vi "Load_Max_Current.vi"(0 "Serial In":refnum<visa-resource-name>, 5 "Node":u8, 7 "Mode":enum16{"Continuous Current", "Peak Current"}(ring), 9 "Max. Current":u16, 11 "Error In":errorcluster) -> (4 "Serial Out":refnum<visa-resource-name>, 15 "Error Out":errorcluster)   [LabVIEW 2019, in "Faulhaber RS232.lvlib"]
uses:
  <instrlib>/Faulhaber RS232/Faulhaber RS232.lvlib
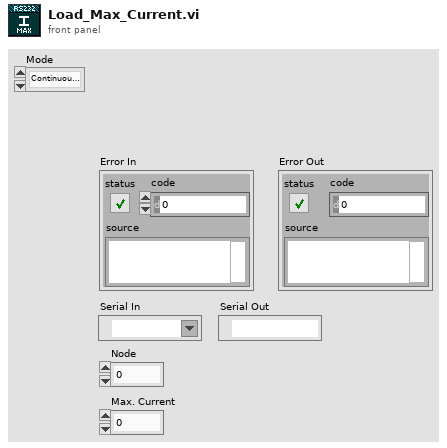
[diagram p1: front panel]
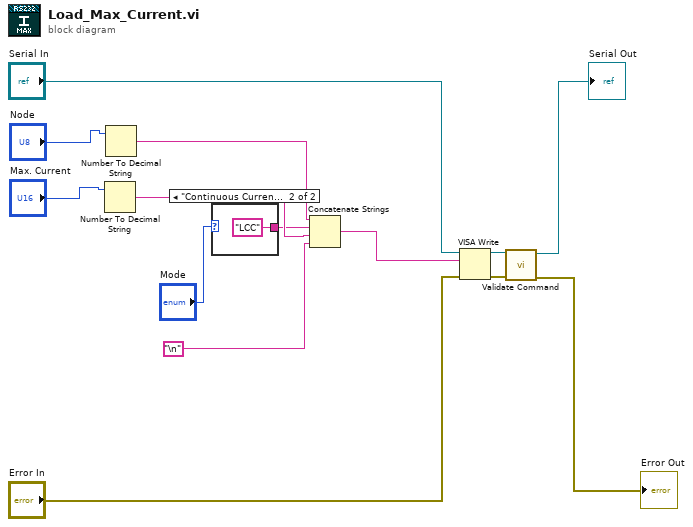
[diagram p0: block diagram]
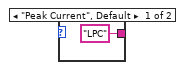
[diagram p2: hidden frame]
diagram:
  n1 = Number To Decimal String(number="Max. Current") -> (decimal integer string=w9:string)  [unwired: 1 in]
  n2 = Number To Decimal String(number="Node") -> (decimal integer string=w10:string)  [unwired: 1 in]
  n3 = case shown="\"Continuous Current\"" "Mode" {
    tunnel: ["LPC" ("string") "LCC" ("string")] -> w7
    frame "Peak Current", Default {
    }
    frame "Continuous Current" {
    }
  }
  n4 = Concatenate Strings(w10, w7, w9, "\n") -> (w8:string)
  n5 = VISA Write(VISA resource name="Serial In", write buffer=w8, error in (no error)="Error In") -> (VISA resource name out=w5:refnum<visa-resource-name>, error out=w4:errorcluster)  [unwired: 1 out]
  n6 = call <instrlib>:"Validate Command.vi"("error in (no error)"=w4, "Serial in"=w5) -> ("error out"=→"Error Out":errorcluster, "Serial Out"=→"Serial Out":refnum<visa-resource-name>)  [unwired: 3 in, 1 out]
